vi "Disabled channel logic 1ch.vi"(7 "reset":bool, 9 "input valid":bool, 11 "U32 data in":u32[](array[numeric])) -> (1 "data ready":bool, 3 "U32 data out":u32[](array[numeric]))   [LabVIEW 2025, in "niUSRP Stream Control (DMA) v1 FPGA.lvclass"]
uses:
  niUSRP Stream Control (DMA) v1 FPGA.lvclass
  niUSRP Stream Control (DMA) v1 FPGA.lvclass/niUSRP Stream Control (DMA) v1 FPGA.ctl
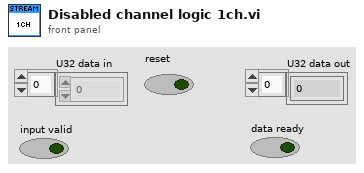
[diagram p1: front panel]
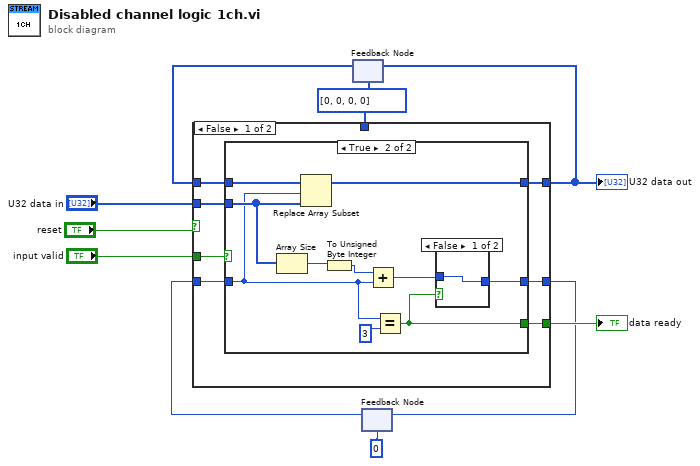
[diagram p0: block diagram]
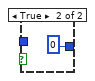
[diagram p3: hidden frame]
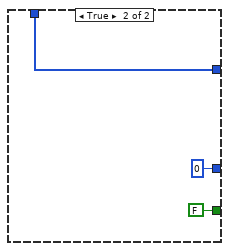
[diagram p4: hidden frame]
diagram:
  w1 = u32[] [0, 0, 0, 0]
  n1 = feedback #1(w1) -> (w5:u32[])
  n2 = feedback #2(u8 0) -> (w4:u8)
  n3 = case shown="False" "reset" {
    tunnel: [w17 FALSE] -> w10
    tunnel: [w16 u8 0] -> w9
    tunnel: [w15 w33] -> w8
    tunnel: "input valid" -> [w14 _]
    tunnel: "U32 data in" -> [w13 _]
    tunnel: w5 -> [w12 _]
    tunnel: w4 -> [w11 _]
    tunnel: w1 -> [_ w33]
    frame False {
      n4 = case shown="True" w14 {
        selector: w14 -> [w18 _]
        tunnel: w13 -> [_ w28]
        tunnel: w11 -> [w20 w24]
        tunnel: [w20 w21] -> w16
        tunnel: w12 -> [w19 w30]
        tunnel: [w19 w29] -> w15
        tunnel: [w18 w23] -> w17
        frame False {
        }
        frame True {
          n5 = Array Size(array=w28) -> (size(s)=w26:i32)
          n6 = Replace Array Subset(array=w30, new element=w28, index=w24) -> (w29:u32[])
          n7 = To Unsigned Byte Integer(number=w26) -> (unsigned 8bit integer=w27:u8)
          n8 = Add(x=w27, y=w24) -> (x+y=w22:u8)
          n9 = Equal?(x=w24, y=u8 3) -> (x = y?=w23:bool)
          n10 = case shown="False" w23 {
            tunnel: [w31 u8 0] -> w21
            tunnel: w22 -> [w31 _]
            frame False {
            }
            frame True {
            }
          }
        }
      }
    }
    frame True {
    }
  }
  "data ready" <- w10
  "U32 data out" <- w8
  n11 = feedback-in #1(w8) -> ()
  n12 = feedback-in #2(w9) -> ()
